vi "Read Anything (from variant).vi"(7 "Type of Anything":variant, 8 "Error In":errorcluster, 9 "Prefix":string, 11 "Variant Database":variant) -> (0 "Error Out":errorcluster, 1 "Found?":bool, 3 "Anything":variant)   [LabVIEW 2020]
doc: "This VI is designed to read data from a file written by <B>Write Anything.vi</B>. If the data type definition has changed since it was written to file, this VI will still read and fill out any elements of the cluster that have the same name. Any elements for which it cannot find a name match in the file will be supplied with their datatype's default value.\n\nFreeware from Moore Good Ideas, www.mooregoodideas.com. Do not remove this line."
uses:
  Koop/KObject Class/KObject.lvclass
  <vilib>/Utility/VariantDataType/VariantType.lvlib
  <vilib>/Utility/Data Type/NI_Data Type.lvlib
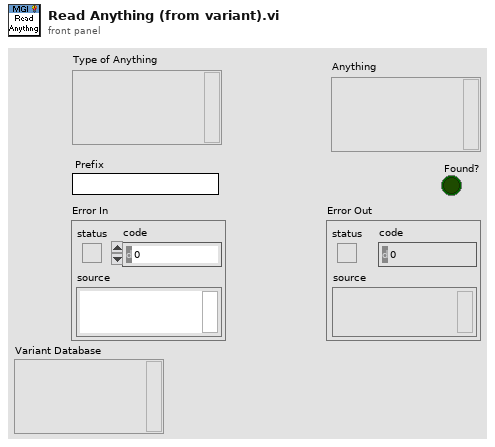
[diagram p1: front panel]
types:
  T1 = typedef "VariantType.lvlib/Type.ctl" = enum8{"Invalid Type", "Void", "I8", "I16", "I32", "I64", "U8", "U16", "U32", "U64", "Single Float", "Double Float", "Extended Float", "Single Complex", "Double Complex", "Extended Complex", "Enum U8", "Enum U16", "Enum U32", "Enum U64", "Single Float With Unit", "Double Float With Unit", "Extended Float With Unit", "Single Complex with Unit", "Double Complex with Unit", "Extended Complex with Unit", "Boolean", "String", "Path", "Picture", "Tag", "Array", "Cluster", "Variant", "LV Variant", "Waveform", "Timestamp", "Digital Waveform", "Digital Data", "ExpressData", "Refnum", "External Data", "VI", "Poly VI", "LabVIEW Class Instance", "Fixed Point"}
  T2 = typedef "NI_Data Type.lvlib/Data Type.ctl" = enum8{"Invalid Type", "Void", "I8", "I16", "I32", "I64", "U8", "U16", "U32", "U64", "Single Float", "Double Float", "Extended Float", "Single Complex", "Double Complex", "Extended Complex", "Enum U8", "Enum U16", "Enum U32", "Enum U64", "Single Float With Unit", "Double Float With Unit", "Extended Float With Unit", "Single Complex with Unit", "Double Complex with Unit", "Extended Complex with Unit", "Boolean", "String", "Path", "Picture", "Tag", "Array", "Cluster", "Variant", "LV Variant", "Waveform", "Timestamp", "Digital Waveform", "Digital Data", "ExpressData", "Refnum", "External Data", "VI", "Poly VI", "LabVIEW Class Instance", "Fixed Point", "Set Collection", "Map Collection"}
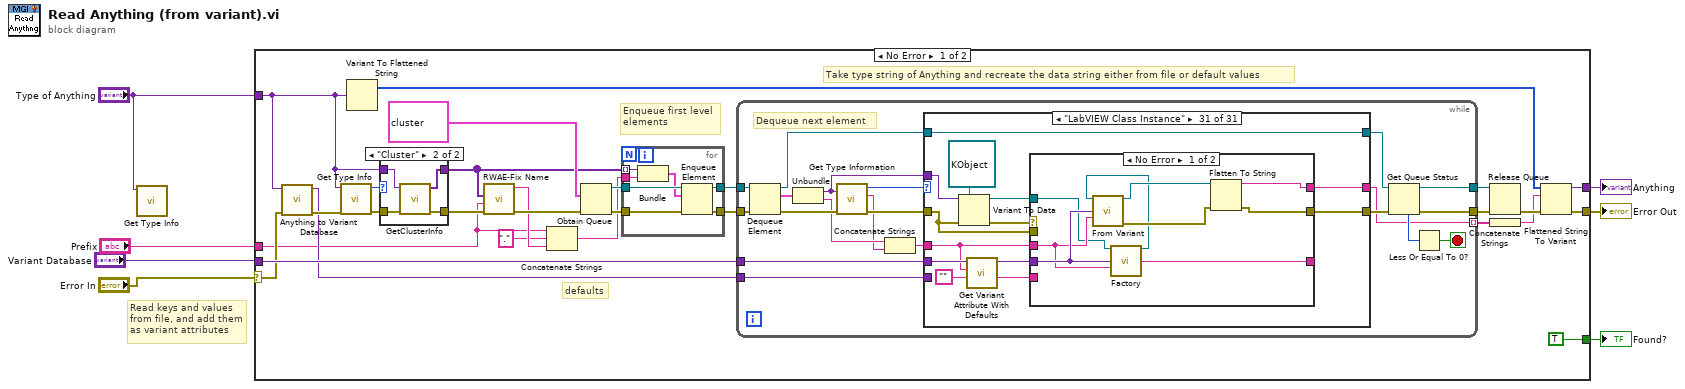
[diagram p0: block diagram]
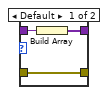
[diagram p2: hidden frame]
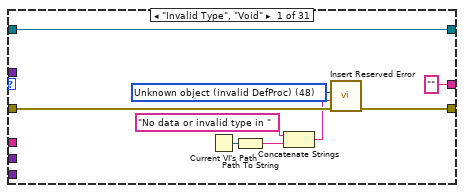
[diagram p3: hidden frame]
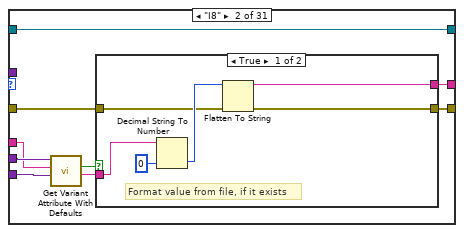
[diagram p4: hidden frame]
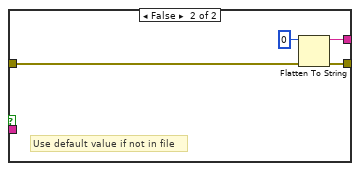
[diagram p5: hidden frame]
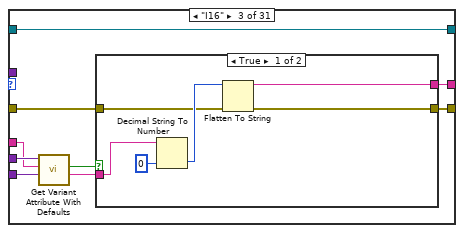
[diagram p6: hidden frame]
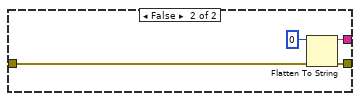
[diagram p7: hidden frame]
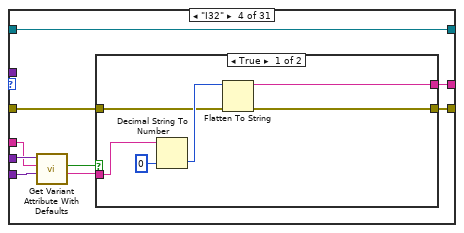
[diagram p8: hidden frame]
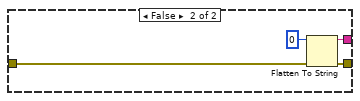
[diagram p9: hidden frame]
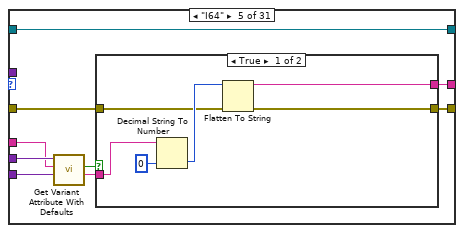
[diagram p10: hidden frame]
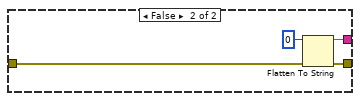
[diagram p11: hidden frame]
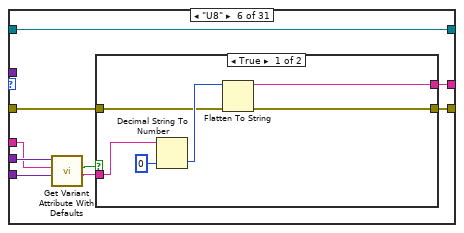
[diagram p12: hidden frame]
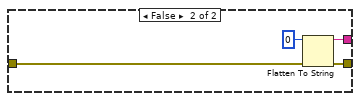
[diagram p13: hidden frame]
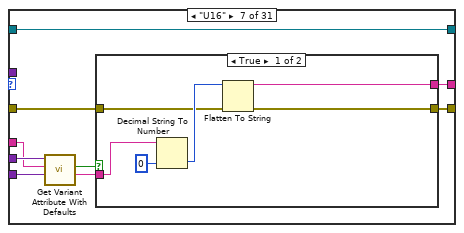
[diagram p14: hidden frame]
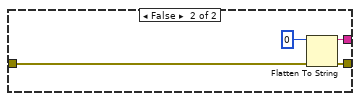
[diagram p15: hidden frame]
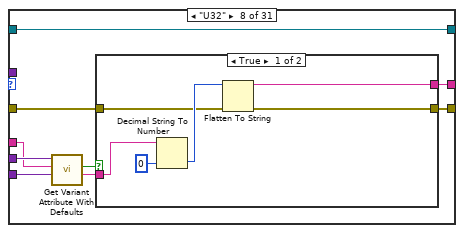
[diagram p16: hidden frame]
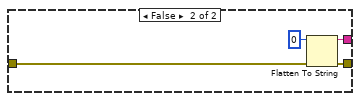
[diagram p17: hidden frame]
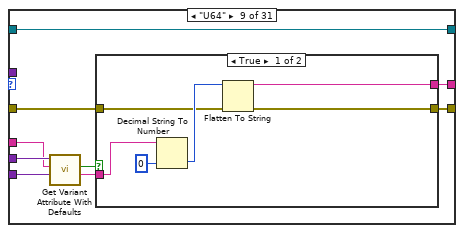
[diagram p18: hidden frame]
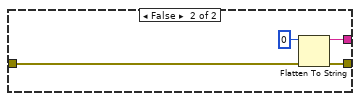
[diagram p19: hidden frame]
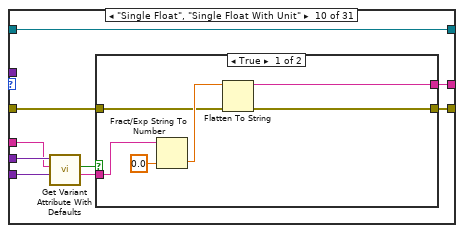
[diagram p20: hidden frame]
diagram:
  # "Read keys and values from file, and add them as variant attributes"
  n1 = call "Get Type Info.vi"("Variant"="Type of Anything") -> ()  [unwired: 8 in, 3 out]
  n2 = case shown="No Error" "Error In" {
    selector: "Error In" -> [w11 w730]
    tunnel: [w34 w730] -> w7
    tunnel: [w33 w732] -> w6
    tunnel: "Type of Anything" -> [w17 w732]
    tunnel: [TRUE FALSE] -> w5
    tunnel: "Variant Database" -> [w21 _]
    tunnel: "Prefix" -> [w9 _]
    frame No Error {
      # "defaults"
      # "Enqueue first level\nelements"
      # "Take type string of Anything and recreate the data string either from file or default values"
      n3 = call "Anything to Variant Database.vi"("Error In"=w11, "Type of Anything"=w17) -> ("Error Out"=w18:errorcluster, "Variant Database"=w16:variant)  [unwired: 8 in]
      n4 = call "Get Type Info.vi"("Error In"=w18, "Variant"=w17) -> ("Error Out"=w19:errorcluster, "Type Enum"=w20:T1)  [unwired: 7 in, 1 out]
      n5 = Variant To Flattened String(Variant=w17) -> (1:w35:i16[])  [unwired: 1 out]
      n6 = case shown="\"Cluster\"" w20 {
        tunnel: [w38 w41] -> w15
        tunnel: w19 -> [w38 w42]
        tunnel: w17 -> [w37 w40]
        tunnel: [w36 w39] -> w13
        frame Default {
          n7 = Build Array(w37) -> (w36:variant[])
        }
        frame "Cluster" {
          n8 = call <vilib>:"GetClusterInfo.vi"("error in (no error)"=w42, "Variant"=w40) -> ("error out"=w41:errorcluster, "Cluster Elements"=w39:variant[])  [unwired: 8 in]
        }
      }
      n9 = call "RWAE-Fix Name.vi"("error in (no error)"=w15, "Section Name (Name of \"Anything\")"=w9, "Cluster Elements in"=w13) -> ("error out"=w14:errorcluster, "Name"=w12:string)  [unwired: 7 in]
      n10 = Concatenate Strings(w9, "." ("string"), w12) -> (w10:string)
      n11 = Obtain Queue(element data type=cluster{"Variant":variant, "Name":string} {"Variant"=variant, "Name"=""}, error in (no error)=w14) -> (queue out=w31:refnum<queue>, error out=w24:errorcluster)  [unwired: 3 in, 1 out]
      n12 = for {
        tunnel: w31 -> [w49]
        tunnel: [w48] -> w30
        tunnel: [w47] -> w29
        tunnel: w13 -> [w46] mode=indexing
        tunnel: w10 -> [w44]
        tunnel: w24 -> [w43]
        n13 = Bundle("ArrayElt"=w46, w44) -> (w45:cluster{"ArrayElt":variant, string})  [unwired: 1 in]
        n14 = Enqueue Element(queue=w49, element=w45, error in (no error)=w43) -> (queue out=w47:refnum<queue>, error out=w48:errorcluster)  [unwired: 1 in, 1 out]
      }
      n15 = while {
        tunnel: w30 -> [w67]
        tunnel: [w62] -> w28
        tunnel: w21 -> [w54]
        tunnel: [w51] -> w32 mode=indexing
        tunnel: w29 -> [w64]
        tunnel: [w58] -> w26
        tunnel: w16 -> [w50]
        stop <- w59 stop-if-true
        # "Dequeue next element"
        n16 = Dequeue Element(queue=w64, error in (no error)=w67) -> (queue out=w65:refnum<queue>, element=w57:cluster{"Variant":variant, "Name":string}, error out=w66:errorcluster)  [unwired: 1 in, 1 out]
        n17 = Unbundle(w57) -> ("Variant"=w53:variant, "Name"=w55:string)
        n18 = call <vilib>:"Get Type Information.vi"("error in (no error)"=w66, "variant"=w53) -> ("error out"=w68:errorcluster, "name"=w52:string, "type"=w69:T2)  [unwired: 5 in, 2 out]
        n19 = Concatenate Strings(w55, w52) -> (w56:string)
        n20 = case shown="\"LabVIEW Class Instance\"" w69 {
          tunnel: [w72 w87 w106 w125 w144 w163 w182 w201 w220 w239 w258 w277 w296 w315 w334 w354 w380 w406 w432 w457 w476 w493 w508 w530 w559 w588 w617 w646 w674 w686 w715] -> w63
          tunnel: w68 -> [w73 w86 w105 w124 w143 w162 w181 w200 w219 w238 w257 w276 w295 w314 w333 w353 w379 w405 w431 w456 w475 w492 w514 w529 w558 w587 w616 w645 w675 w685 w714]
          tunnel: w56 -> [_ w80 w99 w118 w137 w156 w175 w194 w215 w234 w252 w272 w290 w310 w329 w347 w373 w400 w426 w450 w471 w487 w504 w525 w554 w582 w610 w640 w670 w678 w707]
          tunnel: ["" ("data string") w85 w104 w123 w142 w161 w180 w199 w218 w237 w256 w275 w294 w313 w332 w352 w378 w404 w430 w455 w474 w491 "" w528 w557 w586 w615 w644 w672 w684 w716] -> w51
          tunnel: w53 -> [_ _ _ _ _ _ _ _ _ _ _ _ _ _ _ w351 w377 w403 w429 _ _ _ w513 _ _ _ _ _ w673 _ w717]
          tunnel: w65 -> [w74 w84 w103 w122 w141 w160 w179 w198 w217 w236 w255 w274 w293 w312 w331 w350 w376 w402 w428 w454 w473 w490 w509 w527 w556 w585 w614 w643 w677 w683 w719]
          tunnel: [w74 w84 w103 w122 w141 w160 w179 w198 w217 w236 w255 w274 w293 w312 w331 w350 w376 w402 w428 w454 w473 w490 w507 w527 w556 w585 w614 w643 w676 w683 w719] -> w61
          tunnel: w54 -> [_ w81 w100 w119 w138 w157 w176 w195 w216 w235 w253 w273 w291 w311 w330 w349 w374 w401 w427 w451 w472 w488 _ w526 w555 w584 w613 w641 w671 w681 w718]
          tunnel: w50 -> [_ w79 w98 w117 w136 w155 w174 w193 w212 w231 w250 w269 w288 w307 w326 w345 w371 w397 w423 w449 w468 w485 _ w522 w551 w580 w609 w638 w668 _ _]
          frame "Invalid Type", "Void" {
            w70 = u16 48 items=["No error", "Argument error", "Memory is full", "Out of zone", "End of file", "File already open", "Generic file I/O error", "File not found", "File permission error", "Disk is full", "Duplicate path", "Too many files open", "System feature not enabled", "Resource file not found", "Cannot add resource", "Resource not found", "Image not found", "Image memory error", "Pen does not exist", "Config type invalid", "Config token not found", "Config parse error", "Config memory error", "Bad external code format", "Bad external code offset", "External code not present", "Null window", "Destroy window error", "Null menu", "Print aborted", "Bad print record", "Print driver error", "Windows error during printing", "Memory error during printing", "Print dialog error", "Generic print error", "Invalid device refnum", "Device not found", "Device parameter error", "Device unit error", "Cannot open device", "Device call aborted", "Generic error", "Cancelled by user", "Object ID too low", "Object ID too high", "Object not in heap", "Unknown heap", "Unknown object (invalid DefProc)", "Unknown object (DefProc not in table)", "Message out of range", "Invalid (null) method", "Unknown message", "Manager call not supported", "Bad address", "Network operation in progress", "Network operation timed out", "Connection is busy", "Network attribute not supported", "Network error", "Address in use", "System out of memory", "Connection aborted", "Connection refused", "Not connected", "Already connected", "Connection closed", "Initialization error (interapplication manager)", "Bad occurrence", "Wait on unbound occurrence handler", "Occurrence queue overflow", "Datalog type conflict", "Unused", "Unrecognized type (interapplication manager)", "Memory corrupt", "Failed to make temporary DLL", "Old CIN version", "Drag socket not found", "Failed to load drop-object", "Failed to register OLE object", "Failed to release OLE object", "Format specifier type mismatch", "Unknown format specifier", "Too few format specifiers", "Too many format specifiers", "Scan failed", "Newer CIN version", "OLE Convert", "Runtime menu error", "Password tampered", "Unknown error code"] ("Reserved Error Code")
            n21 = Current VI's Path() -> (path=w76:path)
            n22 = Path To String(path=w76) -> (string=w75:string)
            n23 = Concatenate Strings("No data or invalid type in " ("string"), w75) -> (w71:string)
            n24 = call "Insert Reserved Error.vi"("error in (no error)"=w73, "non-standard source (\"\")"=w71, "Reserved Error Code"=w70) -> ("error out"=w72:errorcluster)  [unwired: 4 in]
          }
          frame "I8" {
            n25 = call "Get Variant Attribute With Defaults.vi"("Variant Database defaults"=w79, "name"=w80, "Variant Database from file"=w81) -> ("values"=w82:string, "found"=w83:bool)  [unwired: 6 in, 1 out]
            n26 = case shown="True" w83 {
              tunnel: w82 -> [w88 _]
              tunnel: [w91 w94] -> w87
              tunnel: w86 -> [w90 w95]
              tunnel: [w92 w97] -> w85
              frame True {
                # "Format value from file, if it exists"
                n27 = Decimal String To Number(string=w88, default (0L)=i8 0 ("default (0 I32)")) -> (number=w93:i8)  [unwired: 1 in, 1 out]
                n28 = Flatten To String(anything=w93, error in (no error)=w90) -> (data string=w92:string, error out=w91:errorcluster)  [unwired: 2 in, 1 out]
              }
              frame False {
                # "Use default value if not in file"
                n29 = Flatten To String(anything=i8 0, error in (no error)=w95) -> (data string=w97:string, error out=w94:errorcluster)  [unwired: 2 in, 1 out]
              }
            }
          }
          frame "I16" {
            n30 = call "Get Variant Attribute With Defaults.vi"("Variant Database defaults"=w98, "name"=w99, "Variant Database from file"=w100) -> ("values"=w101:string, "found"=w102:bool)  [unwired: 6 in, 1 out]
            n31 = case shown="True" w102 {
              tunnel: w101 -> [w107 _]
              tunnel: [w110 w113] -> w106
              tunnel: w105 -> [w109 w114]
              tunnel: [w111 w116] -> w104
              frame True {
                n32 = Decimal String To Number(string=w107, default (0L)=i16 0 ("default (0 I32)")) -> (number=w112:i16)  [unwired: 1 in, 1 out]
                n33 = Flatten To String(anything=w112, error in (no error)=w109) -> (data string=w111:string, error out=w110:errorcluster)  [unwired: 2 in, 1 out]
              }
              frame False {
                n34 = Flatten To String(anything=i16 0, error in (no error)=w114) -> (data string=w116:string, error out=w113:errorcluster)  [unwired: 2 in, 1 out]
              }
            }
          }
          frame "I32" {
            n35 = call "Get Variant Attribute With Defaults.vi"("Variant Database defaults"=w117, "name"=w118, "Variant Database from file"=w119) -> ("values"=w120:string, "found"=w121:bool)  [unwired: 6 in, 1 out]
            n36 = case shown="True" w121 {
              tunnel: w120 -> [w126 _]
              tunnel: [w129 w132] -> w125
              tunnel: w124 -> [w128 w133]
              tunnel: [w130 w135] -> w123
              frame True {
                n37 = Decimal String To Number(string=w126, default (0L)=0 ("default (0 I32)")) -> (number=w131:i32)  [unwired: 1 in, 1 out]
                n38 = Flatten To String(anything=w131, error in (no error)=w128) -> (data string=w130:string, error out=w129:errorcluster)  [unwired: 2 in, 1 out]
              }
              frame False {
                n39 = Flatten To String(anything=0, error in (no error)=w133) -> (data string=w135:string, error out=w132:errorcluster)  [unwired: 2 in, 1 out]
              }
            }
          }
          frame "I64" {
            n40 = call "Get Variant Attribute With Defaults.vi"("Variant Database defaults"=w136, "name"=w137, "Variant Database from file"=w138) -> ("values"=w139:string, "found"=w140:bool)  [unwired: 6 in, 1 out]
            n41 = case shown="True" w140 {
              tunnel: w139 -> [w145 _]
              tunnel: [w148 w151] -> w144
              tunnel: w143 -> [w147 w152]
              tunnel: [w149 w154] -> w142
              frame True {
                n42 = Decimal String To Number(string=w145, default (0L)=i64 0 ("default (0 I32)")) -> (number=w150:i64)  [unwired: 1 in, 1 out]
                n43 = Flatten To String(anything=w150, error in (no error)=w147) -> (data string=w149:string, error out=w148:errorcluster)  [unwired: 2 in, 1 out]
              }
              frame False {
                n44 = Flatten To String(anything=i64 0, error in (no error)=w152) -> (data string=w154:string, error out=w151:errorcluster)  [unwired: 2 in, 1 out]
              }
            }
          }
          frame "U8" {
            n45 = call "Get Variant Attribute With Defaults.vi"("Variant Database defaults"=w155, "name"=w156, "Variant Database from file"=w157) -> ("values"=w158:string, "found"=w159:bool)  [unwired: 6 in, 1 out]
            n46 = case shown="True" w159 {
              tunnel: w158 -> [w164 _]
              tunnel: [w167 w170] -> w163
              tunnel: w162 -> [w166 w171]
              tunnel: [w168 w173] -> w161
              frame True {
                n47 = Decimal String To Number(string=w164, default (0L)=u8 0 ("default (0 I32)")) -> (number=w169:u8)  [unwired: 1 in, 1 out]
                n48 = Flatten To String(anything=w169, error in (no error)=w166) -> (data string=w168:string, error out=w167:errorcluster)  [unwired: 2 in, 1 out]
              }
              frame False {
                n49 = Flatten To String(anything=u8 0, error in (no error)=w171) -> (data string=w173:string, error out=w170:errorcluster)  [unwired: 2 in, 1 out]
              }
            }
          }
          frame "U16" {
            n50 = call "Get Variant Attribute With Defaults.vi"("Variant Database defaults"=w174, "name"=w175, "Variant Database from file"=w176) -> ("values"=w177:string, "found"=w178:bool)  [unwired: 6 in, 1 out]
            n51 = case shown="True" w178 {
              tunnel: w177 -> [w183 _]
              tunnel: [w186 w189] -> w182
              tunnel: w181 -> [w185 w190]
              tunnel: [w187 w192] -> w180
              frame True {
                n52 = Decimal String To Number(string=w183, default (0L)=u16 0 ("default (0 I32)")) -> (number=w188:u16)  [unwired: 1 in, 1 out]
                n53 = Flatten To String(anything=w188, error in (no error)=w185) -> (data string=w187:string, error out=w186:errorcluster)  [unwired: 2 in, 1 out]
              }
              frame False {
                n54 = Flatten To String(anything=u16 0, error in (no error)=w190) -> (data string=w192:string, error out=w189:errorcluster)  [unwired: 2 in, 1 out]
              }
            }
          }
          frame "U32" {
            n55 = call "Get Variant Attribute With Defaults.vi"("Variant Database defaults"=w193, "name"=w194, "Variant Database from file"=w195) -> ("values"=w196:string, "found"=w197:bool)  [unwired: 6 in, 1 out]
            n56 = case shown="True" w197 {
              tunnel: w196 -> [w202 _]
              tunnel: [w205 w208] -> w201
              tunnel: w200 -> [w204 w209]
              tunnel: [w206 w211] -> w199
              frame True {
                n57 = Decimal String To Number(string=w202, default (0L)=u32 0 ("default (0 I32)")) -> (number=w207:u32)  [unwired: 1 in, 1 out]
                n58 = Flatten To String(anything=w207, error in (no error)=w204) -> (data string=w206:string, error out=w205:errorcluster)  [unwired: 2 in, 1 out]
              }
              frame False {
                n59 = Flatten To String(anything=u32 0, error in (no error)=w209) -> (data string=w211:string, error out=w208:errorcluster)  [unwired: 2 in, 1 out]
              }
            }
          }
          frame "U64" {
            n60 = call "Get Variant Attribute With Defaults.vi"("Variant Database defaults"=w212, "name"=w215, "Variant Database from file"=w216) -> ("values"=w214:string, "found"=w213:bool)  [unwired: 6 in, 1 out]
            n61 = case shown="True" w213 {
              tunnel: w214 -> [w221 _]
              tunnel: [w224 w227] -> w220
              tunnel: w219 -> [w223 w228]
              tunnel: [w225 w230] -> w218
              frame True {
                n62 = Decimal String To Number(string=w221, default (0L)=u64 0 ("default (0 I32)")) -> (number=w226:u64)  [unwired: 1 in, 1 out]
                n63 = Flatten To String(anything=w226, error in (no error)=w223) -> (data string=w225:string, error out=w224:errorcluster)  [unwired: 2 in, 1 out]
              }
              frame False {
                n64 = Flatten To String(anything=u64 0, error in (no error)=w228) -> (data string=w230:string, error out=w227:errorcluster)  [unwired: 2 in, 1 out]
              }
            }
          }
          frame "Single Float", "Single Float With Unit" {
            n65 = call "Get Variant Attribute With Defaults.vi"("Variant Database defaults"=w231, "name"=w234, "Variant Database from file"=w235) -> ("values"=w233:string, "found"=w232:bool)  [unwired: 6 in, 1 out]
            n66 = case shown="True" w232 {
              tunnel: w233 -> [w240 _]
              tunnel: [w243 w246] -> w239
              tunnel: w238 -> [w242 w247]
              tunnel: [w244 w249] -> w237
              frame True {
                n67 = Fract/Exp String To Number(string=w240, default (0 dbl)=sgl 0.0 ("default (0 I32)")) -> (number=w245:sgl)  [unwired: 2 in, 1 out]
                n68 = Flatten To String(anything=w245, error in (no error)=w242) -> (data string=w244:string, error out=w243:errorcluster)  [unwired: 2 in, 1 out]
              }
              frame False {
                n69 = Flatten To String(anything=sgl 0.0, error in (no error)=w247) -> (data string=w249:string, error out=w246:errorcluster)  [unwired: 2 in, 1 out]
              }
            }
          }
          frame "Double Float", "Double Float With Unit" {
            n70 = call "Get Variant Attribute With Defaults.vi"("Variant Database defaults"=w250, "name"=w252, "Variant Database from file"=w253) -> ("values"=w254:string, "found"=w251:bool)  [unwired: 6 in, 1 out]
            n71 = case shown="True" w251 {
              tunnel: w254 -> [w259 _]
              tunnel: [w262 w265] -> w258
              tunnel: w257 -> [w261 w266]
              tunnel: [w263 w268] -> w256
              frame True {
                n72 = Fract/Exp String To Number(string=w259, default (0 dbl)=0.0 ("default (0 DBL)")) -> (number=w264:dbl)  [unwired: 2 in, 1 out]
                n73 = Flatten To String(anything=w264, error in (no error)=w261) -> (data string=w263:string, error out=w262:errorcluster)  [unwired: 2 in, 1 out]
              }
              frame False {
                n74 = Flatten To String(anything=0.0, error in (no error)=w266) -> (data string=w268:string, error out=w265:errorcluster)  [unwired: 2 in, 1 out]
              }
            }
          }
          frame "Extended Float", "Extended Float With Unit" {
            n75 = call "Get Variant Attribute With Defaults.vi"("Variant Database defaults"=w269, "name"=w272, "Variant Database from file"=w273) -> ("values"=w271:string, "found"=w270:bool)  [unwired: 6 in, 1 out]
            n76 = case shown="True" w270 {
              tunnel: w271 -> [w278 _]
              tunnel: [w281 w284] -> w277
              tunnel: w276 -> [w280 w285]
              tunnel: [w282 w287] -> w275
              frame True {
                n77 = Fract/Exp String To Number(string=w278, default (0 dbl)=ext 0.0 ("default (0 DBL)")) -> (number=w283:ext)  [unwired: 2 in, 1 out]
                n78 = Flatten To String(anything=w283, error in (no error)=w280) -> (data string=w282:string, error out=w281:errorcluster)  [unwired: 2 in, 1 out]
              }
              frame False {
                n79 = Flatten To String(anything=ext 0.0, error in (no error)=w285) -> (data string=w287:string, error out=w284:errorcluster)  [unwired: 2 in, 1 out]
              }
            }
          }
          frame "Single Complex", "Single Complex with Unit" {
            n80 = call "Get Variant Attribute With Defaults.vi"("Variant Database defaults"=w288, "name"=w290, "Variant Database from file"=w291) -> ("values"=w292:string, "found"=w289:bool)  [unwired: 6 in, 1 out]
            n81 = case shown="True" w289 {
              tunnel: w292 -> [w297 _]
              tunnel: [w301 w303] -> w296
              tunnel: w295 -> [w300 w304]
              tunnel: [w302 w306] -> w294
              frame True {
                n82 = Scan From String(input string=w297, default 1=csg 0.0+0.0i ("default (0 DBL)")) -> (output 1=w298:csg)  [unwired: 3 in, 3 out]
                n83 = Flatten To String(anything=w298, error in (no error)=w300) -> (data string=w302:string, error out=w301:errorcluster)  [unwired: 2 in, 1 out]
              }
              frame False {
                n84 = Flatten To String(anything=csg 0.0+0.0i, error in (no error)=w304) -> (data string=w306:string, error out=w303:errorcluster)  [unwired: 2 in, 1 out]
              }
            }
          }
          frame "Double Complex", "Double Complex with Unit" {
            n85 = call "Get Variant Attribute With Defaults.vi"("Variant Database defaults"=w307, "name"=w310, "Variant Database from file"=w311) -> ("values"=w309:string, "found"=w308:bool)  [unwired: 6 in, 1 out]
            n86 = case shown="True" w308 {
              tunnel: w309 -> [w316 _]
              tunnel: [w320 w322] -> w315
              tunnel: w314 -> [w319 w323]
              tunnel: [w321 w325] -> w313
              frame True {
                n87 = Scan From String(input string=w316, default 1=cdb 0.0+0.0i ("default (0 DBL)")) -> (output 1=w318:cdb)  [unwired: 3 in, 3 out]
                n88 = Flatten To String(anything=w318, error in (no error)=w319) -> (data string=w321:string, error out=w320:errorcluster)  [unwired: 2 in, 1 out]
              }
              frame False {
                n89 = Flatten To String(anything=cdb 0.0+0.0i, error in (no error)=w323) -> (data string=w325:string, error out=w322:errorcluster)  [unwired: 2 in, 1 out]
              }
            }
          }
          frame "Extended Complex", "Extended Complex with Unit" {
            n90 = call "Get Variant Attribute With Defaults.vi"("Variant Database defaults"=w326, "name"=w329, "Variant Database from file"=w330) -> ("values"=w328:string, "found"=w327:bool)  [unwired: 6 in, 1 out]
            n91 = case shown="True" w327 {
              tunnel: w328 -> [w335 _]
              tunnel: [w339 w341] -> w334
              tunnel: w333 -> [w338 w342]
              tunnel: [w340 w344] -> w332
              frame True {
                n92 = Scan From String(input string=w335, default 1=cxt 0.0+0.0i ("default (0 DBL)")) -> (output 1=w336:cxt)  [unwired: 3 in, 3 out]
                n93 = Flatten To String(anything=w336, error in (no error)=w338) -> (data string=w340:string, error out=w339:errorcluster)  [unwired: 2 in, 1 out]
              }
              frame False {
                n94 = Flatten To String(anything=cxt 0.0+0.0i, error in (no error)=w342) -> (data string=w344:string, error out=w341:errorcluster)  [unwired: 2 in, 1 out]
              }
            }
          }
          frame "Enum U8" {
            n95 = call "Get Variant Attribute With Defaults.vi"("Variant Database defaults"=w345, "name"=w347, "Variant Database from file"=w349) -> ("values"=w348:string, "found"=w346:bool)  [unwired: 6 in, 1 out]
            n96 = case shown="True" w346 {
              tunnel: w348 -> [w355 _]
              tunnel: [w365 w368] -> w354
              tunnel: w353 -> [w364 w369]
              tunnel: [w366 w370] -> w352
              tunnel: w351 -> [w363 _]
              frame True {
                n97 = call <vilib>:"GetNumericInfo.vi"("error in (no error)"=w364, "Variant"=w363) -> ("error out"=w356:errorcluster, "EnumNames"=w362:string[])  [unwired: 6 in, 2 out]
                n98 = Search 1D Array(1D array=w362, element=w355) -> (index of element=w361:i32)  [unwired: 1 in]
                n99 = In Range and Coerce(upper limit=255, x=w361, lower limit=0) -> (coerced(x)=w359:i32)  [unwired: 1 out]
                n100 = To Unsigned Byte Integer(number=w359) -> (unsigned 8bit integer=w360:u8)
                n101 = Flatten To String(anything=w360, error in (no error)=w356) -> (data string=w366:string, error out=w365:errorcluster)  [unwired: 2 in, 1 out]
              }
              frame False {
                n102 = Flatten To String(anything=u8 0, error in (no error)=w369) -> (data string=w370:string, error out=w368:errorcluster)  [unwired: 2 in, 1 out]
              }
            }
          }
          frame "Enum U16" {
            n103 = call "Get Variant Attribute With Defaults.vi"("Variant Database defaults"=w371, "name"=w373, "Variant Database from file"=w374) -> ("values"=w375:string, "found"=w372:bool)  [unwired: 6 in, 1 out]
            n104 = case shown="True" w372 {
              tunnel: w375 -> [w381 _]
              tunnel: [w391 w394] -> w380
              tunnel: w379 -> [w390 w395]
              tunnel: [w392 w396] -> w378
              tunnel: w377 -> [w389 _]
              frame True {
                n105 = call <vilib>:"GetNumericInfo.vi"("error in (no error)"=w390, "Variant"=w389) -> ("error out"=w382:errorcluster, "EnumNames"=w388:string[])  [unwired: 6 in, 2 out]
                n106 = Search 1D Array(1D array=w388, element=w381) -> (index of element=w387:i32)  [unwired: 1 in]
                n107 = In Range and Coerce(upper limit=u16 65535, x=w387, lower limit=0) -> (coerced(x)=w385:i32)  [unwired: 1 out]
                n108 = To Unsigned Word Integer(number=w385) -> (unsigned 16bit integer=w386:u16)
                n109 = Flatten To String(anything=w386, error in (no error)=w382) -> (data string=w392:string, error out=w391:errorcluster)  [unwired: 2 in, 1 out]
              }
              frame False {
                n110 = Flatten To String(anything=u16 0, error in (no error)=w395) -> (data string=w396:string, error out=w394:errorcluster)  [unwired: 2 in, 1 out]
              }
            }
          }
          frame "Enum U32" {
            n111 = call "Get Variant Attribute With Defaults.vi"("Variant Database defaults"=w397, "name"=w400, "Variant Database from file"=w401) -> ("values"=w399:string, "found"=w398:bool)  [unwired: 6 in, 1 out]
            n112 = case shown="True" w398 {
              tunnel: w399 -> [w407 _]
              tunnel: [w417 w420] -> w406
              tunnel: w405 -> [w416 w421]
              tunnel: [w418 w422] -> w404
              tunnel: w403 -> [w415 _]
              frame True {
                n113 = call <vilib>:"GetNumericInfo.vi"("error in (no error)"=w416, "Variant"=w415) -> ("error out"=w408:errorcluster, "EnumNames"=w414:string[])  [unwired: 6 in, 2 out]
                n114 = Search 1D Array(1D array=w414, element=w407) -> (index of element=w413:i32)  [unwired: 1 in]
                n115 = In Range and Coerce(upper limit=u32 4294967295, x=w413, lower limit=0) -> (coerced(x)=w411:u32)  [unwired: 1 out]
                n116 = To Unsigned Long Integer(number=w411) -> (unsigned 32bit integer=w412:u32)
                n117 = Flatten To String(anything=w412, error in (no error)=w408) -> (data string=w418:string, error out=w417:errorcluster)  [unwired: 2 in, 1 out]
              }
              frame False {
                n118 = Flatten To String(anything=u32 0, error in (no error)=w421) -> (data string=w422:string, error out=w420:errorcluster)  [unwired: 2 in, 1 out]
              }
            }
          }
          frame "Enum U64" {
            n119 = call "Get Variant Attribute With Defaults.vi"("Variant Database defaults"=w423, "name"=w426, "Variant Database from file"=w427) -> ("values"=w425:string, "found"=w424:bool)  [unwired: 6 in, 1 out]
            n120 = case shown="True" w424 {
              tunnel: [w443 w446] -> w432
              tunnel: w431 -> [w442 w447]
              tunnel: [w444 w448] -> w430
              tunnel: w429 -> [w441 _]
              tunnel: w425 -> [w433 _]
              frame True {
                n121 = call <vilib>:"GetNumericInfo.vi"("error in (no error)"=w442, "Variant"=w441) -> ("error out"=w434:errorcluster, "EnumNames"=w440:string[])  [unwired: 6 in, 2 out]
                n122 = Search 1D Array(1D array=w440, element=w433) -> (index of element=w439:i32)  [unwired: 1 in]
                n123 = In Range and Coerce(upper limit=u64 18446744073709551615, x=w439, lower limit=0) -> (coerced(x)=w437:u64)  [unwired: 1 out]
                n124 = To Unsigned Quad Integer(1:w437) -> (0:w438:u64)
                n125 = Flatten To String(anything=w438, error in (no error)=w434) -> (data string=w444:string, error out=w443:errorcluster)  [unwired: 2 in, 1 out]
              }
              frame False {
                n126 = Flatten To String(anything=u64 0, error in (no error)=w447) -> (data string=w448:string, error out=w446:errorcluster)  [unwired: 2 in, 1 out]
              }
            }
          }
          frame "Boolean" {
            n127 = call "Get Variant Attribute With Defaults.vi"("Variant Database defaults"=w449, "name"=w450, "Variant Database from file"=w451) -> ("values"=w452:string, "found"=w453:bool)  [unwired: 6 in, 1 out]
            n128 = case shown="True" w453 {
              tunnel: w452 -> [w458 _]
              tunnel: [w462 w465] -> w457
              tunnel: w456 -> [w459 w466]
              tunnel: [w463 w467] -> w455
              frame True {
                n129 = Equal?(x=w458, y="TRUE") -> (x = y?=w460:bool)
                n130 = Flatten To String(anything=w460, error in (no error)=w459) -> (data string=w463:string, error out=w462:errorcluster)  [unwired: 2 in, 1 out]
              }
              frame False {
                n131 = Flatten To String(anything=FALSE, error in (no error)=w466) -> (data string=w467:string, error out=w465:errorcluster)  [unwired: 2 in, 1 out]
              }
            }
          }
          frame "String" {
            n132 = call "Get Variant Attribute With Defaults.vi"("Variant Database defaults"=w468, "name"=w471, "Variant Database from file"=w472) -> ("values"=w469:string, "found"=w470:bool)  [unwired: 6 in, 1 out]
            n133 = case shown="True" w470 {
              tunnel: [w479 w482] -> w476
              tunnel: w475 -> [w478 w483]
              tunnel: [w480 w484] -> w474
              tunnel: w469 -> [w477 _]
              frame True {
                n134 = Flatten To String(anything=w477, error in (no error)=w478) -> (data string=w480:string, error out=w479:errorcluster)  [unwired: 2 in, 1 out]
              }
              frame False {
                n135 = Flatten To String(anything="", error in (no error)=w483) -> (data string=w484:string, error out=w482:errorcluster)  [unwired: 2 in, 1 out]
              }
            }
          }
          frame "Path" {
            n136 = call "Get Variant Attribute With Defaults.vi"("Variant Database defaults"=w485, "name"=w487, "Variant Database from file"=w488) -> ("values"=w486:string, "found"=w489:bool)  [unwired: 6 in, 1 out]
            n137 = case shown="True" w489 {
              tunnel: [w497 w500] -> w493
              tunnel: w492 -> [w496 w501]
              tunnel: [w498 w502] -> w491
              tunnel: w486 -> [w494 _]
              frame True {
                n138 = String To Path(string=w494) -> (path=w495:path)
                n139 = Flatten To String(anything=w495, error in (no error)=w496) -> (data string=w498:string, error out=w497:errorcluster)  [unwired: 2 in, 1 out]
              }
              frame False {
                n140 = Flatten To String(anything=path "", error in (no error)=w501) -> (data string=w502:string, error out=w500:errorcluster)  [unwired: 2 in, 1 out]
              }
            }
          }
          frame "Cluster" {
            # "Enqueue cluster elements"
            n141 = call <vilib>:"GetClusterInfo.vi"("error in (no error)"=w514, "Variant"=w513) -> ("error out"=w510:errorcluster, "Cluster Elements"=w512:variant[])  [unwired: 8 in]
            n142 = Concatenate Strings(w504, "." ("string")) -> (w503:string)
            n143 = Reverse 1D Array(array=w512) -> (reversed array=w511:variant[])
            n144 = for {
              tunnel: w509 -> [w521]
              tunnel: w510 -> [w520]
              tunnel: [w519] -> w508
              tunnel: [w518] -> w507
              tunnel: w511 -> [w517] mode=indexing
              tunnel: w503 -> [w515]
              n145 = Bundle("ArrayElt"=w517, w515) -> (w516:cluster{"ArrayElt":variant, string})  [unwired: 1 in]
              n146 = Enqueue Element At Opposite End(queue=w521, element=w516, error in (no error)=w520) -> (queue out=w518:refnum<queue>, error out=w519:errorcluster)  [unwired: 1 in, 1 out]
            }
          }
          frame "Variant", "LV Variant" {
            n147 = call "Get Variant Attribute With Defaults.vi"("Variant Database defaults"=w522, "name"=w525, "Variant Database from file"=w526) -> ("values"=w524:string, "found"=w523:bool)  [unwired: 6 in, 1 out]
            n148 = case shown="True" w523 {
              tunnel: w524 -> [w531 _]
              tunnel: [w539 w548] -> w530
              tunnel: w529 -> [w539 w549]
              tunnel: [w537 w550] -> w528
              frame True {
                n149 = String Subset(string=w531, offset (0)=2) -> (substring=w536:string)  [unwired: 1 in]
                n150 = String Length(string=w536) -> (length=w534:i32)
                n151 = Multiply(x=0.5, y=w534) -> (x*y=w533:dbl)
                n152 = for {
                  N: w533 -> [_]
                  tunnel: w536 -> [w543]
                  tunnel: [w545] -> w535 mode=indexing
                  i -> [w542]
                  w541 = 2 ("length (rest)")
                  n153 = Multiply(x=w542, y=w541) -> (x*y=w540:i32)
                  n154 = String Subset(string=w543, offset (0)=w540, length (rest)=w541) -> (substring=w544:string)
                  n155 = Hexadecimal String To Number(string=w544, default (0uL)=u8 0 ("default (0 U32)")) -> (number=w545:u8)  [unwired: 1 in, 1 out]
                }
                n156 = Byte Array To String(unsigned byte array=w535) -> (string=w537:string)
              }
              frame False {
                w547 = variant  # Variant
                n157 = Flatten To String(anything=w547, error in (no error)=w549) -> (data string=w550:string, error out=w548:errorcluster)  [unwired: 2 in, 1 out]
              }
            }
          }
          frame "Waveform" {
            n158 = call "Get Variant Attribute With Defaults.vi"("Variant Database defaults"=w551, "name"=w554, "Variant Database from file"=w555) -> ("values"=w553:string, "found"=w552:bool)  [unwired: 6 in, 1 out]
            n159 = case shown="False" w552 {
              tunnel: w553 -> [w560 _]
              tunnel: [w568 w578] -> w559
              tunnel: w558 -> [w568 w577]
              tunnel: [w566 w579] -> w557
              frame True {
                n160 = String Subset(string=w560, offset (0)=2) -> (substring=w565:string)  [unwired: 1 in]
                n161 = String Length(string=w565) -> (length=w563:i32)
                n162 = Multiply(x=0.5, y=w563) -> (x*y=w562:dbl)
                n163 = for {
                  N: w562 -> [_]
                  tunnel: w565 -> [w572]
                  tunnel: [w574] -> w564 mode=indexing
                  i -> [w571]
                  w570 = 2 ("length (rest)")
                  n164 = Multiply(x=w571, y=w570) -> (x*y=w569:i32)
                  n165 = String Subset(string=w572, offset (0)=w569, length (rest)=w570) -> (substring=w573:string)
                  n166 = Hexadecimal String To Number(string=w573, default (0uL)=u8 0 ("default (0 U32)")) -> (number=w574:u8)  [unwired: 1 in, 1 out]
                }
                n167 = Byte Array To String(unsigned byte array=w564) -> (string=w566:string)
              }
              frame False {
                n168 = Flatten To String(anything=waveform(dbl) {"t0"=timestamp(0 s since 1904-01-01), "dt"=0.0, "Y"=[]} ("Waveform 2"), error in (no error)=w577) -> (data string=w579:string, error out=w578:errorcluster)  [unwired: 2 in, 1 out]
              }
            }
          }
          frame "Timestamp" {
            n169 = call "Get Variant Attribute With Defaults.vi"("Variant Database defaults"=w580, "name"=w582, "Variant Database from file"=w584) -> ("values"=w583:string, "found"=w581:bool)  [unwired: 6 in, 1 out]
            n170 = case shown="False" w581 {
              tunnel: w583 -> [w589 _]
              tunnel: [w597 w607] -> w588
              tunnel: w587 -> [w597 w606]
              tunnel: [w595 w608] -> w586
              frame True {
                n171 = String Subset(string=w589, offset (0)=2) -> (substring=w594:string)  [unwired: 1 in]
                n172 = String Length(string=w594) -> (length=w592:i32)
                n173 = Multiply(x=0.5, y=w592) -> (x*y=w591:dbl)
                n174 = for {
                  N: w591 -> [_]
                  tunnel: w594 -> [w601]
                  tunnel: [w603] -> w593 mode=indexing
                  i -> [w600]
                  w599 = 2 ("length (rest)")
                  n175 = Multiply(x=w600, y=w599) -> (x*y=w598:i32)
                  n176 = String Subset(string=w601, offset (0)=w598, length (rest)=w599) -> (substring=w602:string)
                  n177 = Hexadecimal String To Number(string=w602, default (0uL)=u8 0 ("default (0 U32)")) -> (number=w603:u8)  [unwired: 1 in, 1 out]
                }
                n178 = Byte Array To String(unsigned byte array=w593) -> (string=w595:string)
              }
              frame False {
                n179 = Flatten To String(anything=timestamp(0 s since 1904-01-01), error in (no error)=w606) -> (data string=w608:string, error out=w607:errorcluster)  [unwired: 2 in, 1 out]
              }
            }
          }
          frame "Digital Waveform" {
            n180 = call "Get Variant Attribute With Defaults.vi"("Variant Database defaults"=w609, "name"=w610, "Variant Database from file"=w613) -> ("values"=w612:string, "found"=w611:bool)  [unwired: 6 in, 1 out]
            n181 = case shown="False" w611 {
              tunnel: w612 -> [w618 _]
              tunnel: [w626 w636] -> w617
              tunnel: w616 -> [w626 w635]
              tunnel: [w624 w637] -> w615
              frame True {
                n182 = String Subset(string=w618, offset (0)=2) -> (substring=w623:string)  [unwired: 1 in]
                n183 = String Length(string=w623) -> (length=w621:i32)
                n184 = Multiply(x=0.5, y=w621) -> (x*y=w620:dbl)
                n185 = for {
                  N: w620 -> [_]
                  tunnel: w623 -> [w630]
                  tunnel: [w632] -> w622 mode=indexing
                  i -> [w629]
                  w628 = 2 ("length (rest)")
                  n186 = Multiply(x=w629, y=w628) -> (x*y=w627:i32)
                  n187 = String Subset(string=w630, offset (0)=w627, length (rest)=w628) -> (substring=w631:string)
                  n188 = Hexadecimal String To Number(string=w631, default (0uL)=u8 0 ("default (0 U32)")) -> (number=w632:u8)  [unwired: 1 in, 1 out]
                }
                n189 = Byte Array To String(unsigned byte array=w622) -> (string=w624:string)
              }
              frame False {
                n190 = call <vilib>:"DWDT Empty Digital.vi"() -> ("digital waveform out"=w634:digitalwaveform)  [unwired: 5 in]
                n191 = Flatten To String(anything=w634, error in (no error)=w635) -> (data string=w637:string, error out=w636:errorcluster)  [unwired: 2 in, 1 out]
              }
            }
          }
          frame "Digital Data" {
            n192 = call "Get Variant Attribute With Defaults.vi"("Variant Database defaults"=w638, "name"=w640, "Variant Database from file"=w641) -> ("values"=w642:string, "found"=w639:bool)  [unwired: 6 in, 1 out]
            n193 = case shown="True" w639 {
              tunnel: w642 -> [w647 _]
              tunnel: [w655 w665] -> w646
              tunnel: w645 -> [w655 w664]
              tunnel: [w653 w666] -> w644
              frame True {
                n194 = String Subset(string=w647, offset (0)=2) -> (substring=w652:string)  [unwired: 1 in]
                n195 = String Length(string=w652) -> (length=w650:i32)
                n196 = Multiply(x=0.5, y=w650) -> (x*y=w649:dbl)
                n197 = for {
                  N: w649 -> [_]
                  tunnel: w652 -> [w659]
                  tunnel: [w661] -> w651 mode=indexing
                  i -> [w658]
                  w657 = 2 ("length (rest)")
                  n198 = Multiply(x=w658, y=w657) -> (x*y=w656:i32)
                  n199 = String Subset(string=w659, offset (0)=w656, length (rest)=w657) -> (substring=w660:string)
                  n200 = Hexadecimal String To Number(string=w660, default (0uL)=u8 0 ("default (0 U32)")) -> (number=w661:u8)  [unwired: 1 in, 1 out]
                }
                n201 = Byte Array To String(unsigned byte array=w651) -> (string=w653:string)
              }
              frame False {
                n202 = call <vilib>:"DTbl Empty Digital.vi"() -> ("digital data"=w663:digitaldata)  [unwired: 5 in]
                n203 = Flatten To String(anything=w663, error in (no error)=w664) -> (data string=w666:string, error out=w665:errorcluster)  [unwired: 2 in, 1 out]
              }
            }
          }
          frame "Array" {
            n204 = call "Get Variant Attribute With Defaults.vi"("Variant Database defaults"=w668, "name"=w670, "Variant Database from file"=w671) -> ("values"=w669:string, "Variant out"=w667:variant)  [unwired: 6 in, 1 out]
            n205 = call "Unprocess Array Elements.vi"("Variant Database"=w667, "Value"=w669, "Error In"=w675, "Name In"=w670, "Array Variant"=w673, "Queue In"=w677) -> ("Error Out"=w674:errorcluster, "Data Out"=w672:string, "Queue Out"=w676:refnum<queue>)  [unwired: 3 in]
          }
          frame Default {
            n206 = call "Get Variant Attribute With Defaults.vi"("Variant Database defaults"="", "name"=w678, "Variant Database from file"=w681) -> ("values"=w680:string, "found"=w679:bool)  [unwired: 6 in, 1 out]
            n207 = case shown="True" w679 {
              tunnel: w680 -> [w687 _]
              tunnel: [w695 w704] -> w686
              tunnel: w685 -> [w695 w705]
              tunnel: [w693 w706] -> w684
              frame True {
                n208 = String Subset(string=w687, offset (0)=2) -> (substring=w692:string)  [unwired: 1 in]
                n209 = String Length(string=w692) -> (length=w690:i32)
                n210 = Multiply(x=0.5, y=w690) -> (x*y=w688:dbl)
                n211 = for {
                  N: w688 -> [_]
                  tunnel: w692 -> [w699]
                  tunnel: [w701] -> w691 mode=indexing
                  i -> [w698]
                  w697 = 2 ("length (rest)")
                  n212 = Multiply(x=w698, y=w697) -> (x*y=w696:i32)
                  n213 = String Subset(string=w699, offset (0)=w696, length (rest)=w697) -> (substring=w700:string)
                  n214 = Hexadecimal String To Number(string=w700, default (0uL)=u8 0 ("default (0 U32)")) -> (number=w701:u8)  [unwired: 1 in, 1 out]
                }
                n215 = Byte Array To String(unsigned byte array=w691) -> (string=w693:string)
              }
              frame False {
                n216 = Flatten To String(anything="", error in (no error)=w705) -> (data string=w706:string, error out=w704:errorcluster)  [unwired: 2 in, 1 out]
              }
            }
          }
          frame "LabVIEW Class Instance" {
            n217 = Variant To Data(error in=w714, type=refnum<class "KObject.lvclass"> refnum ("KObject"), Variant=w717) -> (data=w709:refnum<class "KObject.lvclass">, error out=w710:errorcluster)
            n218 = call "Get Variant Attribute With Defaults.vi"("Variant Database defaults"="", "name"=w707, "Variant Database from file"=w718) -> ("values"=w711:string, "Variant out"=w708:variant)  [unwired: 6 in, 1 out]
            n219 = case shown="No Error" w710 {
              tunnel: w711 -> [_ _]
              tunnel: w709 -> [w722 _]
              tunnel: [w726 _] -> w716
              tunnel: [w727 w729] -> w715
              tunnel: w714 -> [_ w729]
              tunnel: w708 -> [w725 _]
              tunnel: w707 -> [w724 _]
              tunnel: [w723 _] -> _
              frame No Error {
                n220 = call-dynamic "Factory.vi"("KObject in"=w722, "Variant"=w725, "Prefix"=w724) -> ("KObject out"=w720:refnum<class "KObject.lvclass">, "Type"=w723:string)  [unwired: 10 in, 1 out]
                n221 = call-dynamic "From Variant.vi"("KObject in"=w720, "Variant"=w725, "Prefix"=w724) -> ("KObject out"=w721:refnum<class "KObject.lvclass">, "error out"=w728:errorcluster)  [unwired: 11 in]
                n222 = Flatten To String(anything=w721, error in (no error)=w728) -> (data string=w726:string, error out=w727:errorcluster)  [unwired: 2 in, 1 out]
              }
              frame Error {
              }
            }
          }
        }
        n223 = Get Queue Status(queue=w61, error in (no error)=w63) -> (queue out=w58:refnum<queue>, error out=w62:errorcluster, # elements in queue=w60:i32)  [unwired: 1 in, 5 out]
        n224 = Less Or Equal To 0?(x=w60) -> (x <= 0?=w59:bool)
      }
      n225 = Release Queue(queue=w26, error in (no error)=w28) -> (error out=w27:errorcluster)  [unwired: 1 in, 2 out]
      n226 = Concatenate Strings(w32) -> (w22:string)
      n227 = Flattened String To Variant(4:w27, 6:w22, 7:w35) -> (0:w34:errorcluster, 3:w33:variant)
    }
    frame Error {
    }
  }
  "Error Out" <- w7
  "Anything" <- w6
  "Found?" <- w5
